vi "SetTempAndWaitSub.vi"(0 "mode (0)":i16, 1 "address string":string, 2 "Heizspannung (V)":dbl, 3 "error in":errorcluster, 4 "Wartezeit zw. Temperaturmessungen":dbl) -> (5 "error out":errorcluster)   [LabVIEW 2010]
uses:
  <vilib>/Analysis/NI_AALBase.lvlib
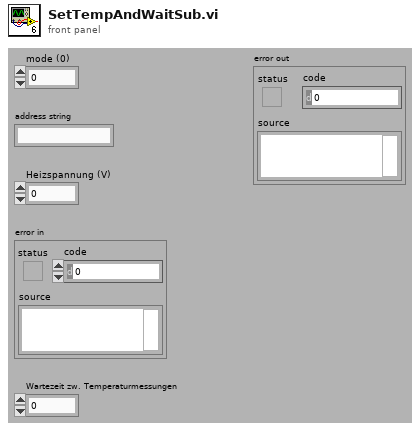
[diagram p1: front panel]
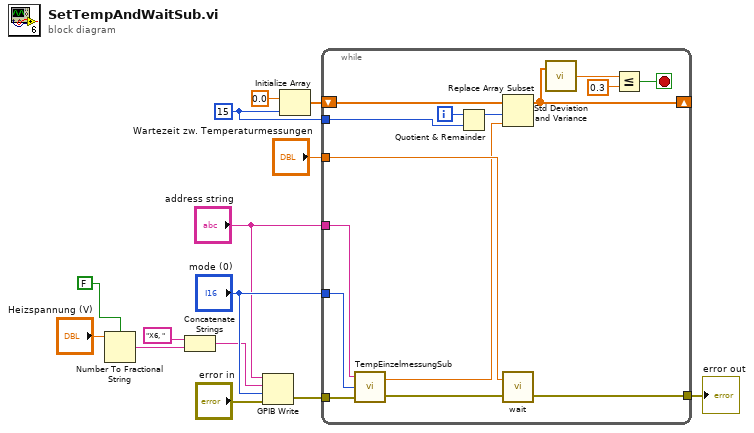
[diagram p0: block diagram]
diagram:
  w14 = 15
  n1 = Number To Fractional String(use system decimal point (T)=FALSE, number="Heizspannung (V)") -> (F-format string=w3:string)  [unwired: 2 in]
  n2 = Concatenate Strings("X6, ", w3) -> (w2:string)
  n3 = GPIB Write(0:"address string", 1:w2, 2:"mode (0)", 3:"error in") -> (6:w7:errorcluster)  [unwired: 1 in, 1 out]
  n4 = Initialize Array(0.0, w14) -> (w13:dbl[])
  n5 = while {
    tunnel: w7 -> [w28]
    tunnel: [w27] -> w8
    tunnel: "address string" -> [w26]
    tunnel: "mode (0)" -> [w25]
    tunnel: "Wartezeit zw. Temperaturmessungen" -> [w24]
    shift-right: [w18] -> _
    shift-left: w13 -> [w22]
    tunnel: w14 -> [w20]
    i -> [w21]
    stop <- w17 stop-if-true
    n6 = call "TempEinzelmessungSub.vi"("error in"=w28, "mode (0)"=w25, "address string"=w26) -> ("error out"=w29:errorcluster, "Numeric"=w23:dbl)
    n7 = Quotient & Remainder(x=w21, y=w20) -> (x-y*floor(x/y)=w16:i32)  [unwired: 1 out]
    n8 = Replace Array Subset(array=w22, new element=w23, index=w16) -> (w18:dbl[])
    n9 = call "wait.vi"("error in"=w29, "Wartezeit in Sek"=w24) -> ("error out"=w27:errorcluster)  [unwired: 1 in]
    n10 = call <vilib>:"Std Deviation and Variance.vi"("X"=w18) -> ("standard deviation"=w15:dbl)  [unwired: 1 in, 2 out]
    n11 = Less Or Equal?(x=w15, y=0.3) -> (x <= y?=w17:bool)
  }
  "error out" <- w8
